vi "Write Delay Line.vi"(10 "Delay Line.lvlib:Abstract Delay Line.lvclass":refnum<class "Abstract Delay Line.lvclass">, 11 "Acquisition Controller in":refnum<class "Acquisition Controller.lvclass">) -> (3 "Acquisition Controller out":refnum<class "Acquisition Controller.lvclass">)   [LabVIEW 2016, in "Controllers.lvlib" / "Acquisition Controller.lvclass"]
uses:
  Acquisition Controller.lvclass
  Delay Line/Abstract Delay Line/Abstract Delay Line.lvclass
  Acquisition Controller.lvclass/Acquisition Controller.ctl
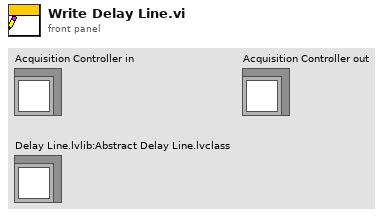
[diagram p1: front panel]
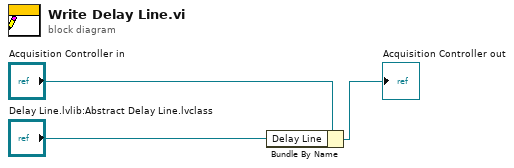
[diagram p0: block diagram]
diagram:
  n1 = Bundle By Name(cluster="Acquisition Controller in", "Delay Line"="Delay Line.lvlib:Abstract Delay Line.lvclass") -> (→"Acquisition Controller out":refnum<class "Acquisition Controller.lvclass">)
